vi "Refresh.vi"(8 "error in (no error)":errorcluster, 11 "Windows System SAL in":refnum<class "Windows System SAL.lvclass">) -> (0 "error out":errorcluster, 3 "Windows System SAL out":refnum<class "Windows System SAL.lvclass">)   [LabVIEW 2020, in "Volatus.lvlib" / "Windows System SAL.lvclass"]
uses:
  Windows System SAL.lvclass
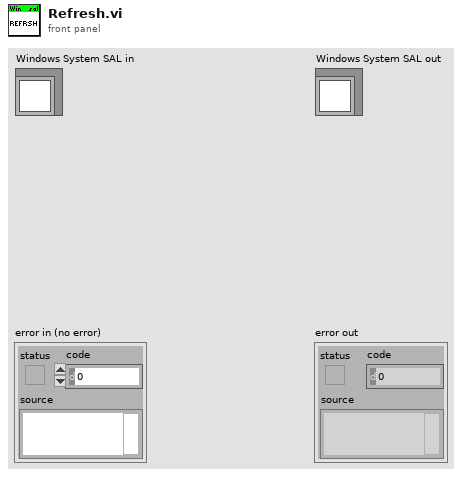
[diagram p1: front panel]
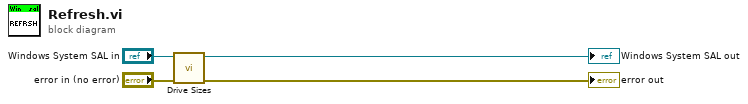
[diagram p0: block diagram]
diagram:
  n1 = call "Drive Sizes.vi"("error in (no error)"="error in (no error)", "Windows System SAL in"="Windows System SAL in") -> ("error out"=→"error out":errorcluster, "Windows System SAL out"=→"Windows System SAL out":refnum<class "Windows System SAL.lvclass">)  [unwired: 8 in]
